vi "gaussian_kernel.vi"(10 "N":i32, 11 "Sigma":dbl) -> (3 "Gaussian kernel":dbl[][](array[numeric]))   [LabVIEW 2022 SP3]
doc: "Generate Gaussian kernel of dimension NxN for given sigma."
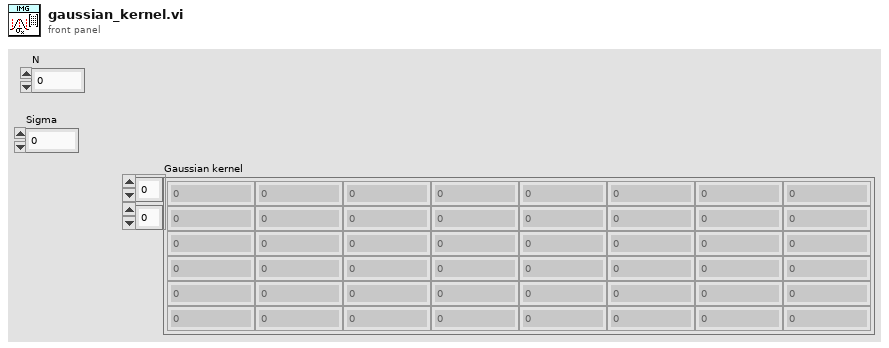
[diagram p1: front panel]
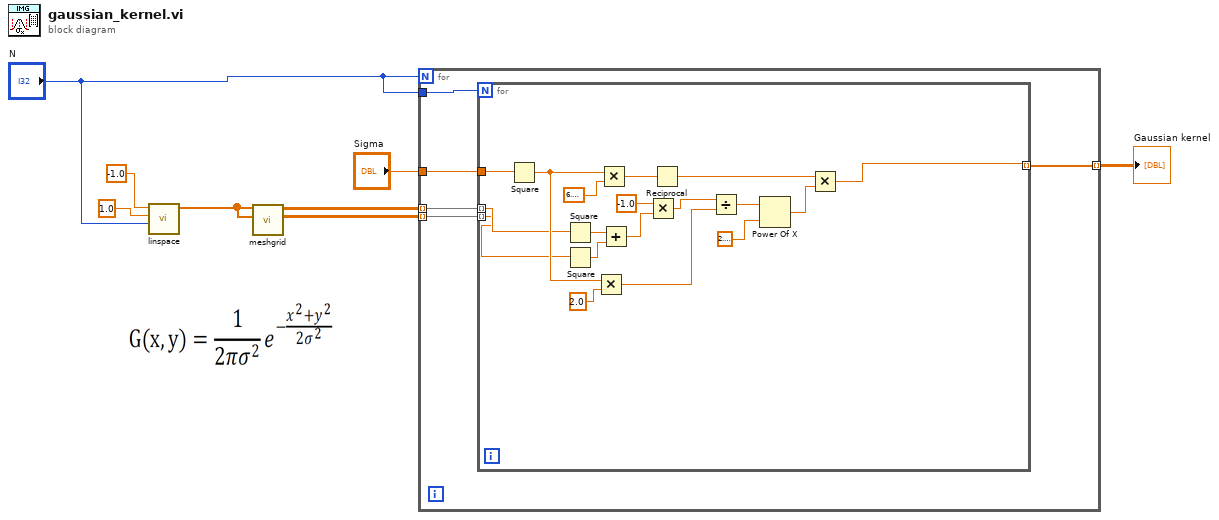
[diagram p0: block diagram]
diagram:
  n1 = call "linspace.vi"("Samples"="N", "Stop"=1.0, "Start"=-1.0) -> ("Array"=w4:dbl[])  [unwired: 8 in]
  n2 = call "meshgrid.vi"("Y in"=w4, "X in"=w4) -> ("Y"=w2:dbl[][], "X"=w3:dbl[][])  [unwired: 8 in]
  n3 = for {
    N: "N" -> [_]
    tunnel: "N" -> [w13]
    tunnel: "Sigma" -> [w12]
    tunnel: w3 -> [w11] mode=indexing
    tunnel: w2 -> [w10] mode=indexing
    tunnel: [w9] -> w1 mode=indexing
    n4 = for {
      N: w13 -> [_]
      tunnel: w12 -> [w25]
      tunnel: w11 -> [w19] mode=indexing
      tunnel: w10 -> [w18] mode=indexing
      tunnel: [w17] -> w9 mode=indexing
      n5 = Square(x=w25) -> (x^2=w24:dbl)
      n6 = Square(x=w19) -> (x^2=w21:dbl)
      n7 = Square(x=w18) -> (x^2=w20:dbl)
      n8 = Multiply(x=w24, y=2.0) -> (x*y=w23:dbl)
      n9 = Multiply(x=w24, y=6.283185307179586) -> (x*y=w30:dbl)
      n10 = Add(x=w21, y=w20) -> (x+y=w16:dbl)
      n11 = Multiply(x=-1.0, y=w16) -> (x*y=w14:dbl)
      n12 = Reciprocal(x=w30) -> (1/x=w29:dbl)
      n13 = Divide(x=w14, y=w23) -> (x/y=w15:dbl)
      n14 = Power Of X(1:2.718281828459045, 2:w15) -> (0:w27:dbl)
      n15 = Multiply(x=w29, y=w27) -> (x*y=w17:dbl)
    }
  }
  "Gaussian kernel" <- w1
